vi "measure_max_power_stabilisation_keithley-2400.vi"(0 "User Name":string, 1 "Cell details cluster":T2={"Cell Position"=16, "Cell Label"="", "Pixel to measure"=0, "Area (cm^2)"=0.126, "Variable"="", "Variable value"="", "Scan settings in queue"=0, "Light or dark"="", "Measurement Type"=""} {"Pixel to measure" items=["All", "1", "2", "3", "4", "5", "6", "7", "8"]}, 3 "Date array":string[](array[string]), 5 "Experiment Title":string, 9 "File path of JV log":path, 11 "Intensity (no. of suns)":string, 12 "Scan settings":T1={"J-V scan"=TRUE, "Start voltage (V)"=0.0, "End voltage (V)"=0.0, "Step voltage (V)"=1.4, "Scan both directions"=TRUE, "Inverted device structure"=FALSE, "Settling delay (ms)"=10.0, "Measurement speed"=0, "Scan rate (V/s)"=0.0, "Stabilisation time (s)"=0.0, "Stabilisation mode"=0, "Stabilisation value (V or A) "=1.0, "Illumination"=0, "Stabilisation in the dark?"=FALSE, "Repeat light scans"=FALSE, "No. of repeat scans"=0.0, "Only repeat for best pixel"=1, "J-t scan"=FALSE, "J-t best pixel only"=7, "J-t start voltage (V)"=0.0, "J-t end voltage (V)"=1.4, "J-t step voltage (V)"=0.01, "Step time (s)"=0.7, "J-t scan both directions"=TRUE, "J-t inverted device structure"=FALSE, "J-t settling delay (ms)"=0.0, "J-t measurement speed"=0, "J-t illumination"=2, "Max. power stabilisation"=FALSE, "Max power best pixel only"=1, "Max. power point tracker"=FALSE, "Vmp from J-V scan"=FALSE, "Max P stab. Specific voltage"=FALSE, "Vmp (V)"=1.0, "Stabilisation time step (s)"=1.0, "Total stabilisation time (s)"=100.0} {"J-t settling delay (ms)" min=10.0; "J-t illumination" items=["Light only", "Dark only", "Light then dark", "Dark then light"]; "Measurement speed" items=["Fast", "Normal", "High accuracy"]; "Illumination" items=["Light only", "Dark only", "Light then dark", "Dark then light"]; "Only repeat for best pixel" items=["only for best pixel", "for best 2 pixels", "for best 3 pixels", "for best 4 pixels", "for best 5 pixels", "for best 6 pixels", "for best 7 pixels", "for all pixels"]; "No. of repeat scans" min=1.0 step=1.0; "Max power best pixel only" items=["only the best pixel", "the best 2 pixels", "the best 3 pixels", "the best 4 pixels", "the best 5 pixels", "the best 6 pixels", "the best 7 pixels", "all pixels"]; "J-t best pixel only" items=["only the best pixel", "the best 2 pixels", "the best 3 pixels", "the best 4 pixels", "the best 5 pixels", "the best 6 pixels", "the best 7 pixels", "all pixels"]; "J-t measurement speed" items=["Fast", "Normal", "High Accuracy"]; "Stabilisation mode" items=["V", "I"]; "Settling delay (ms)" min=10.0}, 13 "VISA resource name":refnum<visa-resource-name>="GPIB1::24::INSTR", 14 "Skip pixel?":bool) -> (4 "Jt Curve":cluster{"Y":dbl[], "Y":dbl[]}[](graph) caption="JV Curve")   [LabVIEW 2016]
uses:
  TypeDefs/scan_settings.ctl
  <vilib>/Utility/file.llb/Read Delimited Spreadsheet (DBL).vi
  <instrlib>/Keithley 24XX/Keithley 24XX.lvlib
panel:
  out "File path for Jt image":path
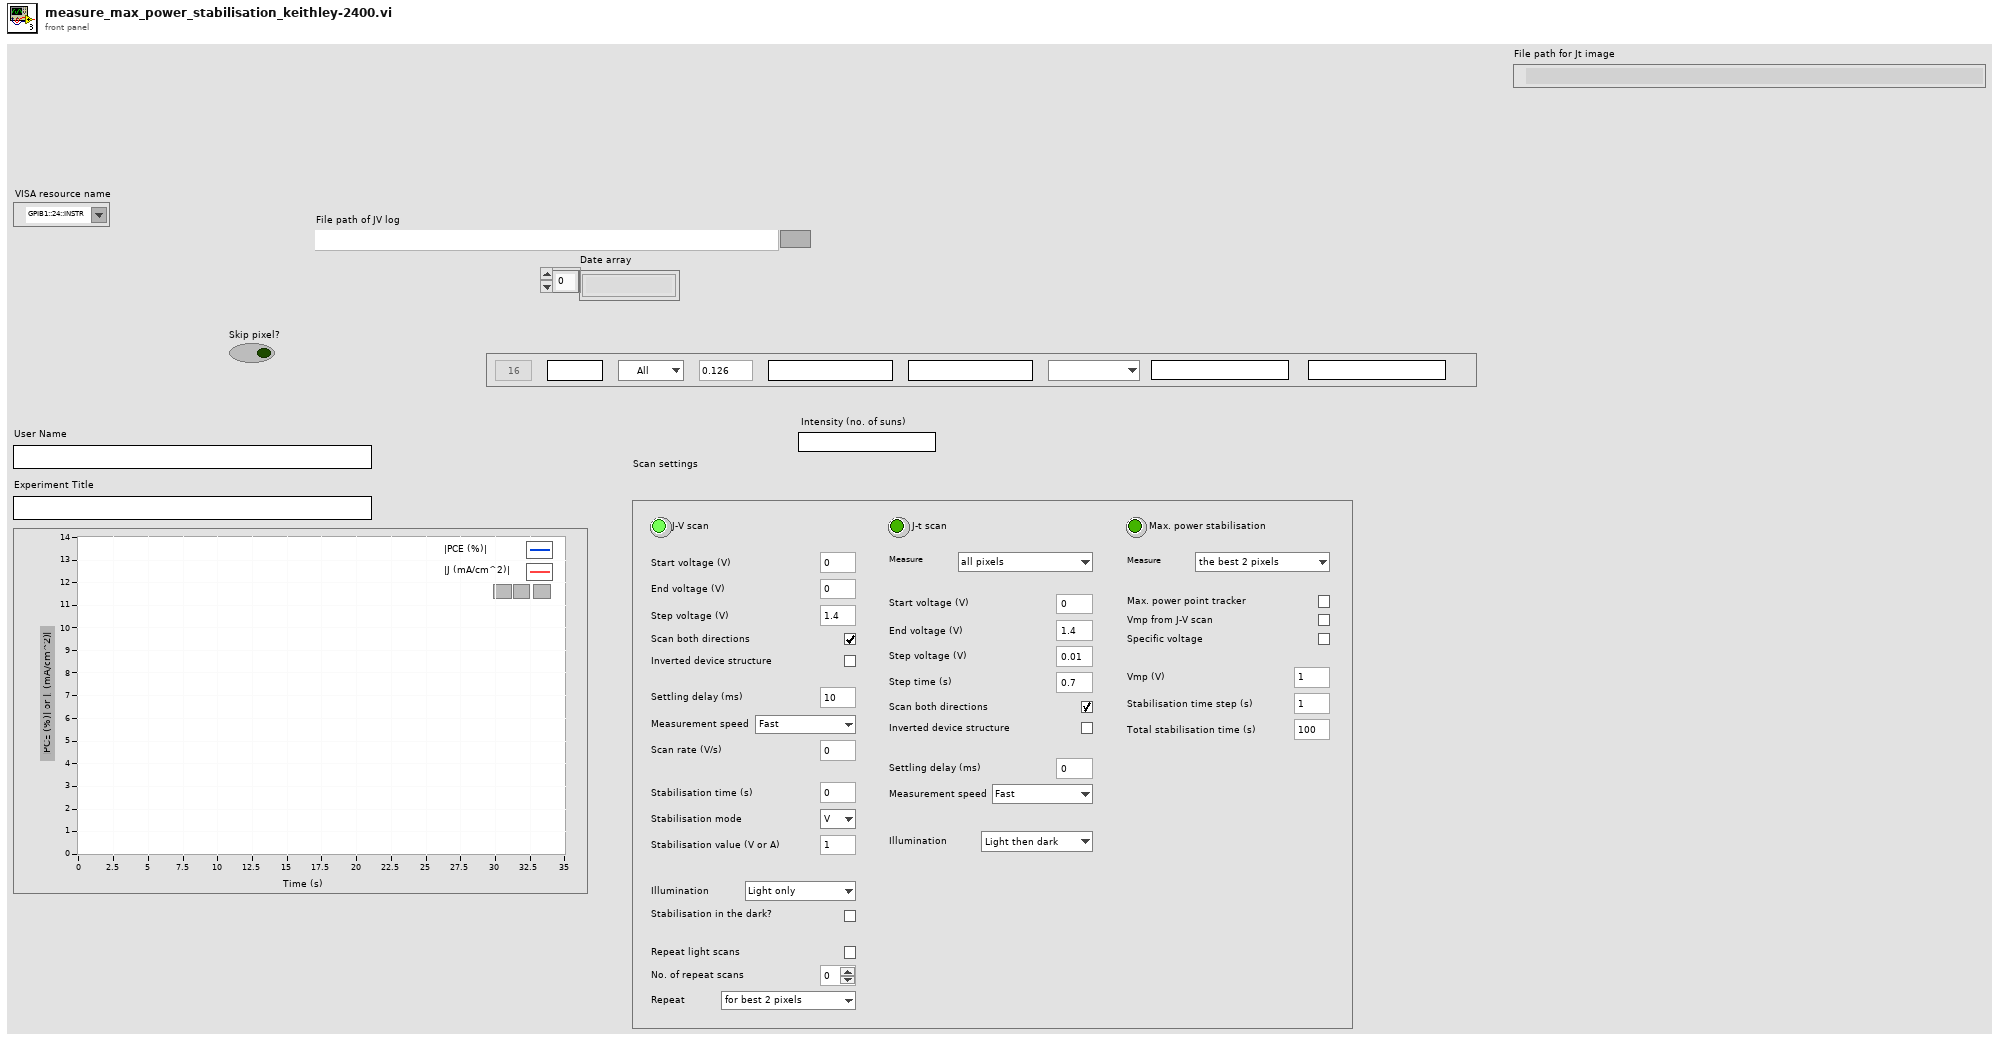
[diagram p1: front panel]
types:
  T1 = typedef "scan_settings.ctl" = cluster{"J-V scan":bool, "Start voltage (V)":dbl, "End voltage (V)":dbl, "Step voltage (V)":dbl, "Scan both directions":bool, "Inverted device structure":bool, "Settling delay (ms)":dbl, "Measurement speed":u8, "Scan rate (V/s)":dbl, "Stabilisation time (s)":dbl, "Stabilisation mode":u16, "Stabilisation value (V or A) ":dbl, "Illumination":u16, "Stabilisation in the dark?":bool, "Repeat light scans":bool, "No. of repeat scans":dbl, "Only repeat for best pixel":u16, "J-t scan":bool, "J-t best pixel only":u16, "J-t start voltage (V)":dbl, "J-t end voltage (V)":dbl, "J-t step voltage (V)":dbl, "Step time (s)":dbl, "J-t scan both directions":bool, "J-t inverted device structure":bool, "J-t settling delay (ms)":dbl, "J-t measurement speed":u16, "J-t illumination":u16, "Max. power stabilisation":bool, "Max power best pixel only":u16, "Max. power point tracker":bool, "Vmp from J-V scan":bool, "Max P stab. Specific voltage":bool, "Vmp (V)":dbl, "Stabilisation time step (s)":dbl, "Total stabilisation time (s)":dbl}
  T2 = cluster{"Cell Position":i32, "Cell Label":string, "Pixel to measure":u16, "Area (cm^2)":dbl, "Variable":string, "Variable value":string, "Scan settings in queue":u16, "Light or dark":string, "Measurement Type":string}
  T3 = typedef "imagedata.ctl" = cluster{"image type":i32, "image depth":i32, "image":u8[], "mask":u8[], "colors":u32[], "Rectangle":cluster{"left":i16, "top":i16, "right":i16, "bottom":i16}}
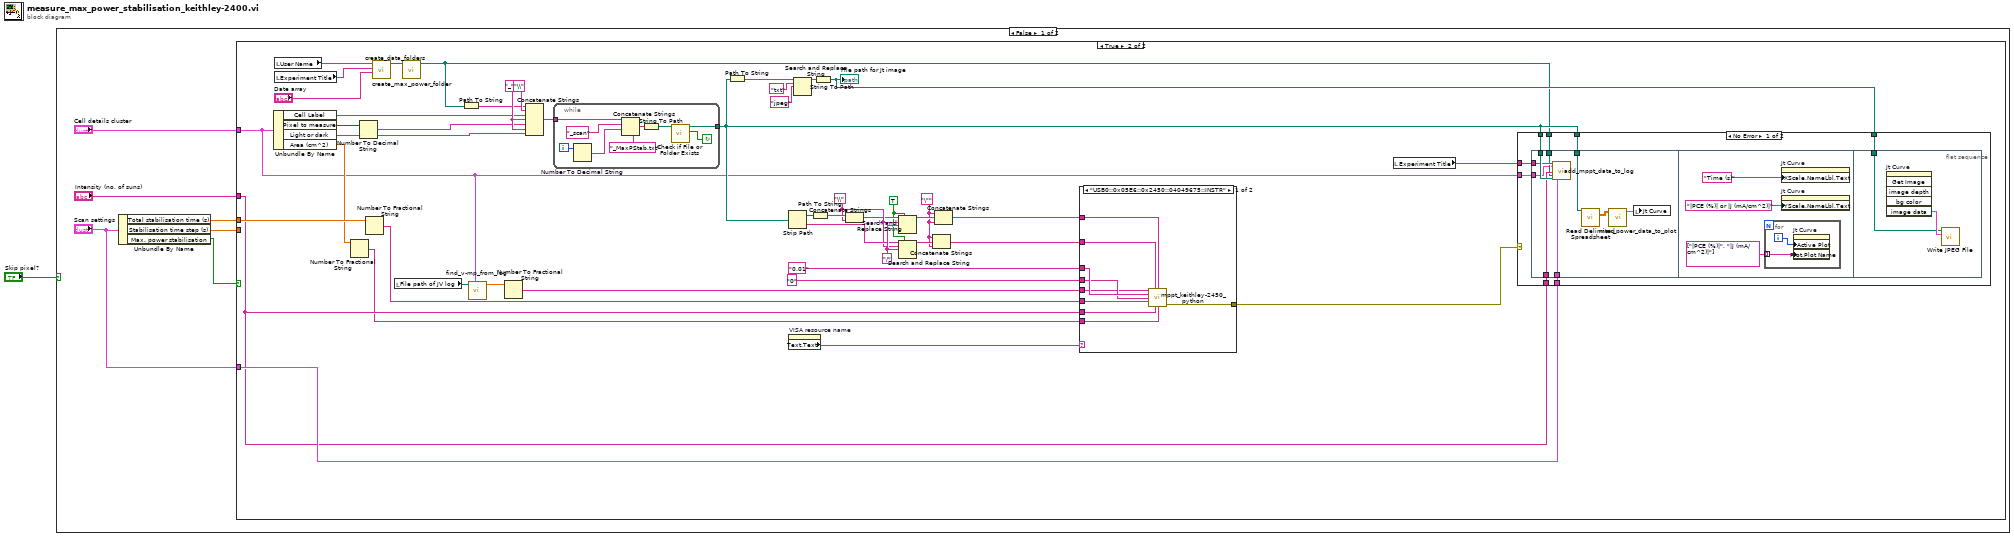
[diagram p0: block diagram]
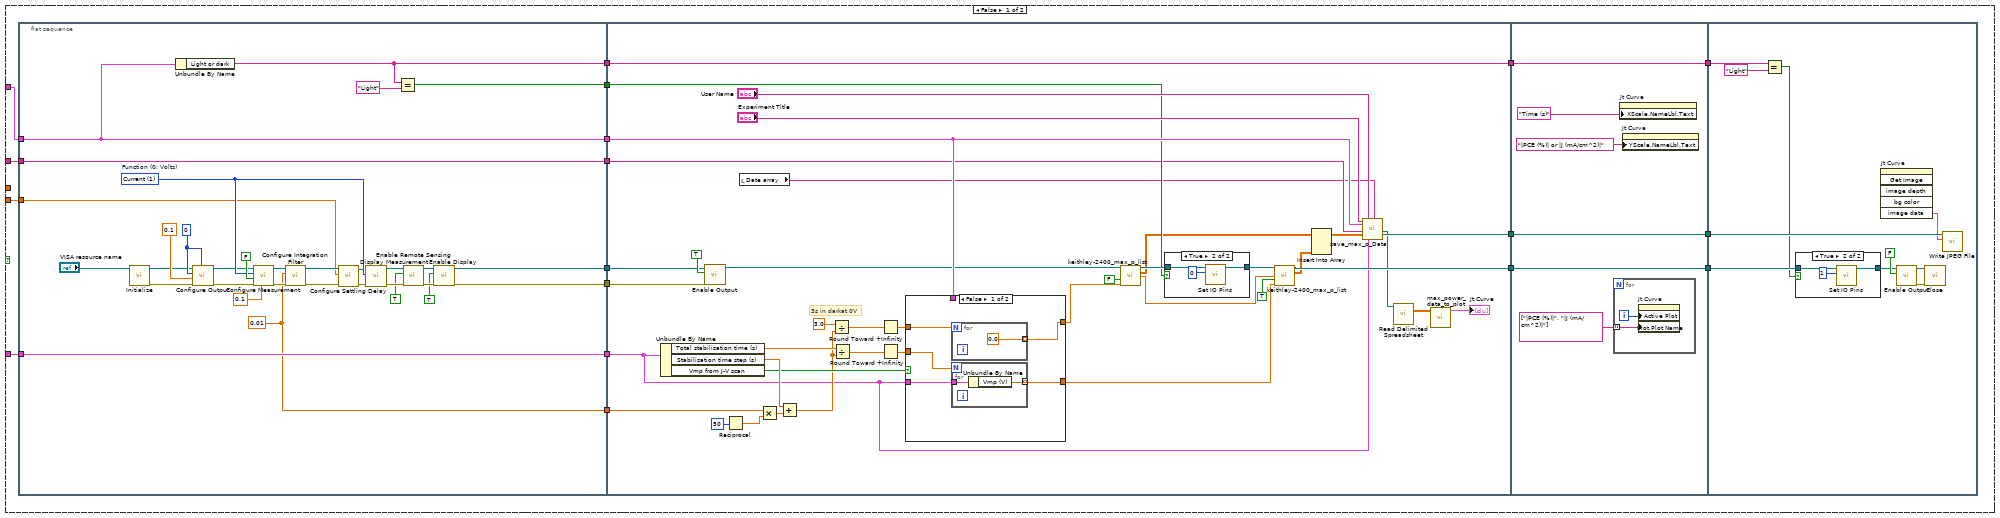
[diagram p2: hidden frame]
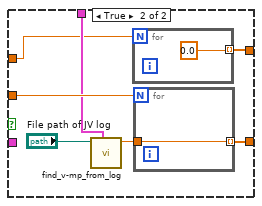
[diagram p4: hidden frame]
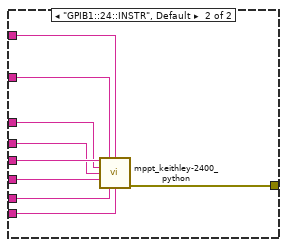
[diagram p6: hidden frame]
diagram:
  n1 = case shown="False" "Skip pixel?" {
    frame False {
      n2 = Unbundle By Name("Scan settings") -> ("Total stabilisation time (s)"=w3:dbl, "Stabilisation time step (s)"=w7:dbl, "Max. power stabilisation"=w4:bool)
      n3 = case shown="True" w4 {
        tunnel: w7 -> [w18 _]
        tunnel: "Cell details cluster" -> [w17 w155]
        tunnel: "Scan settings" -> [w16 w159]
        tunnel: w3 -> [_ w167]
        tunnel: "Intensity (no. of suns)" -> [w14 w151]
        frame False {
          n4 = flat-sequence {
            tunnel: [w35] -> w24
            tunnel: [w36] -> w25
            tunnel: [w37] -> w23
            tunnel: w18 -> [w38]
            tunnel: [w40] -> w22
            tunnel: w17 -> [w40]
            tunnel: [w42] -> w21
            tunnel: w16 -> [w42]
            tunnel: [w39] -> w20
            tunnel: [w34] -> w19
            tunnel: [w26] -> w15
            tunnel: w14 -> [w26]
            tunnel: [w95] -> w13
            tunnel: [w97] -> w11
            tunnel: w25 -> [w64]
            tunnel: w24 -> [w63]
            tunnel: w23 -> [w88]
            tunnel: w22 -> [w81]
            tunnel: w21 -> [w58]
            tunnel: [w91] -> w9
            tunnel: w20 -> [w91]
            tunnel: w19 -> [w68]
            tunnel: w15 -> [w62]
            tunnel: w13 -> [w124]
            tunnel: [w124] -> w12
            tunnel: w11 -> [w123]
            tunnel: [w123] -> w10
            tunnel: w9 -> [w122]
            tunnel: [w122] -> w8
            tunnel: w12 -> [w130]
            tunnel: w10 -> [w133]
            tunnel: w8 -> [w127]
            frame #0 {
              w32 = 0
              w37 = 0.01
              w48 = u16 1 items=["Volts", "Current", "Resistance"]  # Function (0: Volts)
              n5 = call <instrlib>:"Initialize.vi"("VISA resource name"="VISA resource name") -> ("error out"=w27:errorcluster, "VISA resource name out"=w30:refnum<visa-resource-name>)  [unwired: 4 in, 5 out]
              n6 = Unbundle By Name(w40) -> ("Light or dark"=w39:string)
              n7 = call <instrlib>:"Configure Output.vi"("Source Mode  (0: Voltage)"=w32, "error in (no error)"=w27, "Compliance  Level (0.1)"=0.1, "Output Level (0)"=w32, "VISA resource name"=w30) -> ("error out"=w28:errorcluster, "VISA resource name out"=w29:refnum<visa-resource-name>)  [unwired: 5 in]
              n8 = call <instrlib>:"Configure Measurement.vi"("Manual Range (1.0)"=0.1, "error in (no error)"=w28, "Enable Auto Range (T:Enable)"=FALSE, "Function (0: Volts)"=w48, "VISA resource name"=w29) -> ("error out"=w53:errorcluster, "VISA resource name out"=w52:refnum<visa-resource-name>)  [unwired: 5 in]
              n9 = call <instrlib>:"Configure Integration Filter.vi"("error in (no error)"=w53, "Measurement Speed (1 PLC)"=w37, "VISA resource name"=w52) -> ("error out"=w43:errorcluster, "VISA resource name out"=w46:refnum<visa-resource-name>)  [unwired: 7 in]
              n10 = call <instrlib>:"Configure Settling Delay.vi"("error in (no error)"=w43, "Manual Settling Delay (0 sec)"=w38, "VISA resource name"=w46) -> ("error out"=w44:errorcluster, "VISA resource name out"=w45:refnum<visa-resource-name>)  [unwired: 7 in]
              n11 = call <instrlib>:"Display Measurement.vi"("error in (no error)"=w44, "Displayed Measurement (0: Voltage)"=w48, "VISA resource name"=w45) -> ("error out"=w55:errorcluster, "VISA resource name out"=w54:refnum<visa-resource-name>)  [unwired: 7 in]
              n12 = Equal?(x=w39, y="Light") -> (x = y?=w34:bool)
              n13 = call <instrlib>:"Enable Remote Sensing.vi"("error in (no error)"=w55, "Enable Remote Sensing (T: Enable)"=TRUE ("Enable Output (T: Enable)"), "VISA resource name"=w54) -> ("error out"=w50:errorcluster, "VISA resource name out"=w51:refnum<visa-resource-name>)  [unwired: 7 in]
              n14 = call <instrlib>:"Enable Display.vi"("error in (no error)"=w50, "Enable Display (T: Enable)"=TRUE ("Enable Output (T: Enable)"), "VISA resource name"=w51) -> ("error out"=w35:errorcluster, "VISA resource name out"=w36:refnum<visa-resource-name>)  [unwired: 7 in]
            }
            frame #1 {
              # "3s in darkat 0V"
              n15 = Unbundle By Name(w58) -> ("Total stabilisation time (s)"=w85:dbl, "Stabilisation time step (s)"=w86:dbl, "Vmp from J-V scan"=w82:bool)
              n16 = call <instrlib>:"Enable Output.vi"("error in (no error)"=w63, "Enable Output (T: Enable)"=TRUE ("Output (Off)"), "VISA resource name"=w64) -> ("VISA resource name out"=w73:refnum<visa-resource-name>)  [unwired: 7 in, 1 out]
              n17 = Reciprocal(x=50) -> (1/x=w90:dbl)
              n18 = local read "Date array"() -> (w59:string[])
              n19 = Multiply(x=w88, y=w90) -> (x*y=w87:dbl)
              n20 = Add(x=w86, y=w87) -> (x+y=w80:dbl)
              n21 = Divide(x=3.0, y=w80) -> (x/y=w77:dbl)
              n22 = Divide(x=w85, y=w80) -> (x/y=w78:dbl)
              n23 = Round Toward +Infinity(x=w77) -> (ceil(x): smallest int >= x=w76:dbl)
              n24 = Round Toward +Infinity(x=w78) -> (ceil(x): smallest int >= x=w84:dbl)
              n25 = case shown="False" w82 {
                tunnel: w84 -> [w106 w115]
                tunnel: w58 -> [w104 _]
                tunnel: [w105 w114] -> w83
                tunnel: w81 -> [_ w113]
                tunnel: w76 -> [w103 w112]
                tunnel: [w102 w111] -> w74
                frame False {
                  n26 = for {
                    N: w103 -> [_]
                    tunnel: [0.0 ("Vmp")] -> w102 mode=indexing
                  }
                  n27 = for {
                    N: w106 -> [_]
                    tunnel: w104 -> [w109]
                    tunnel: [w108] -> w105 mode=indexing
                    n28 = Unbundle By Name(w109) -> ("Vmp (V)"=w108:dbl)
                  }
                }
                frame True {
                  n29 = call "find_v-mp_from_log.vi"("Cell details cluster in"=w113, "File path of JV log"="File path of JV log") -> ("Vmp"=w110:dbl)  [unwired: 9 in]
                  n30 = for {
                    N: w112 -> [_]
                    tunnel: [0.0 ("Vmp")] -> w111 mode=indexing
                  }
                  n31 = for {
                    N: w115 -> [_]
                    tunnel: [w118] -> w114 mode=indexing
                    tunnel: w110 -> [w118]
                  }
                }
              }
              n32 = call "keithley-2400_max_p_list.vi"("VISA resource name in"=w73, "Light?"=FALSE, "Voltage List"=w74) -> ("VISA resource name out"=w70:refnum<visa-resource-name>, "Data Array"=w67:dbl[][], "timestamp"=w69:sgl)  [unwired: 9 in, 1 out]
              n33 = case shown="True" w68 {
                tunnel: w70 -> [w98 w100]
                tunnel: [w98 w99] -> w75
                frame False {
                }
                frame True {
                  n34 = call <instrlib>:"Set IO Pins.vi"("Output Pattern (0)"=0, "VISA resource name"=w100) -> ("VISA resource name out"=w99:refnum<visa-resource-name>)  [unwired: 8 in, 1 out]
                }
              }
              n35 = call "keithley-2400_max_p_list.vi"("VISA resource name in"=w75, "t=0 timestamp"=w69, "Light?"=TRUE, "Voltage List"=w83) -> ("VISA resource name out"=w95:refnum<visa-resource-name>, "Data Array"=w66:dbl[][])  [unwired: 8 in, 2 out]
              n36 = Insert Into Array(array=w67, new element=w66) -> (w65:dbl[][])  [unwired: 2 in]
              n37 = call "save_max_p_Data.vi"("Experiment Indicator"="Experiment Title", "Cell details cluster"=w81, "Intensity (no. of suns)"=w62, "Data Array"=w65, "Username"="User Name", "Scan settings"=w58, "Date array"=w59) -> ("File path for Jt data"=w61:path, "File path for Jt image"=w97:path)  [unwired: 9 in, 2 out]
              n38 = call-poly <vilib>:"Read Delimited Spreadsheet.vi"("file path (dialog if empty)"=w61) -> ("all rows"=w60:dbl[][])  [unwired: 9 in, 5 out]
              n39 = call "max_power_data_to_plot.vi"("Data Array"=w60) -> ("JV Curve"=→"Jt Curve":cluster{"Y":dbl[], "Y":dbl[]}[])  [unwired: 10 in]
            }
            frame #2 {
              n40 = for {
                tunnel: string[] ["|PCE (%)|", "|J (mA/cm^2)|"] ("Measurement queue") -> [w125] mode=indexing
                i -> [w126]
                n41 = property on="Jt Curve" class="XYGraph (strict)"("Active Plot"=w126, "Plot.Plot Name"=w125) -> ()  [unwired: 2 in, 2 out]
              }
              n42 = property on="Jt Curve" class="XYGraph (strict)"("XScale.NameLbl.Text"="Time (s)" ("Y Scale.Name Label.Text")) -> ()  [unwired: 2 in, 2 out]
              n43 = property on="Jt Curve" class="XYGraph (strict)"("YScale.NameLbl.Text"="|PCE (%)| or |J (mA/cm^2)|" ("Y Scale.Name Label.Text")) -> ()  [unwired: 2 in, 2 out]
            }
            frame #3 {
              n44 = Equal?(x=w127, y="Light") -> (x = y?=w128:bool)
              n45 = case shown="True" w128 {
                tunnel: w130 -> [w137 w139]
                tunnel: [w137 w138] -> w129
                frame False {
                }
                frame True {
                  n46 = call <instrlib>:"Set IO Pins.vi"("Output Pattern (0)"=1, "VISA resource name"=w139) -> ("VISA resource name out"=w138:refnum<visa-resource-name>)  [unwired: 8 in, 1 out]
                }
              }
              n47 = invoke on="Jt Curve" class="XYGraph (strict)" method="Get Image"() -> ("image data"=w132:T3)  [unwired: 6 in, 5 out]
              n48 = call <instrlib>:"Enable Output.vi"("Enable Output (T: Enable)"=FALSE ("Output (Off)"), "VISA resource name"=w129) -> ("error out"=w135:errorcluster, "VISA resource name out"=w136:refnum<visa-resource-name>)  [unwired: 8 in]
              n49 = call <instrlib>:"Close.vi"("error in (no error)"=w135, "VISA resource name"=w136) -> ()  [unwired: 9 in, 1 out]
              n50 = call <vilib>:"Write JPEG File.vi"("image data"=w132, "path to JPEG file"=w133) -> ()  [unwired: 8 in, 2 out]
            }
          }
        }
        frame True {
          w154 = "\"" ("string")
          w142 = TRUE ("replace all? (F)")
          w170 = "/" ("search string")
          w153 = "\\" ("search string")
          w179 = "_"
          n51 = Unbundle By Name(w155) -> ("Cell Label"=w175:string, "Pixel to measure"=w176:u16, "Light or dark"=w173:string, "Area (cm^2)"=w164:dbl)
          n52 = local read "User Name"() -> (w181:string)
          n53 = local read "Experiment Title"() -> (w182:string)
          n54 = Number To Fractional String(number=w164) -> (F-format string=w150:string)  [unwired: 3 in]
          n55 = Number To Decimal String(number=w176) -> (decimal integer string=w174:string)  [unwired: 1 in]
          n56 = Number To Fractional String(number=w167) -> (F-format string=w149:string)  [unwired: 3 in]
          n57 = call "create_data_folders.vi"("Date array"="Date array", "Experiment Indicator"=w182, "username"=w181) -> ("Data Output Folder"=w180:path)  [unwired: 8 in]
          n58 = local read "File path of JV log"() -> (w166:path)
          n59 = call "create_max_power_folder.vi"("Data Folder In"=w180) -> ("Data Output Folder"=w156:path)  [unwired: 10 in]
          n60 = Path To String(path=w156) -> (string=w171:string)
          n61 = call "find_v-mp_from_log.vi"("Cell details cluster in"=w155, "File path of JV log"=w166) -> ("Vmp"=w165:dbl)  [unwired: 9 in]
          n62 = Number To Fractional String(number=w165) -> (F-format string=w148:string)  [unwired: 3 in]
          n63 = Concatenate Strings(w171, "\\", w175, w179, w174, w179, w173) -> (w178:string)
          n64 = while {
            tunnel: w178 -> [w237]
            tunnel: [w229] -> w158
            i -> [w235]
            stop <- w230 continue-if-true
            n65 = Number To Decimal String(number=w235) -> (decimal integer string=w234:string)  [unwired: 1 in]
            n66 = Concatenate Strings(w237, "_scan", w234, "_MaxPStab.txt") -> (w231:string)
            n67 = String To Path(string=w231) -> (path=w232:path)
            n68 = call <vilib>:"Check if File or Folder Exists.vi"("path"=w232) -> ("file or folder exists?"=w230:bool, "dup path"=w229:path)  [unwired: 8 in, 1 out]
          }
          n69 = Path To String(path=w158) -> (string=w186:string)
          n70 = Strip Path(path=w158) -> (stripped path=w162:path, name=w163:string)
          n71 = property on="VISA resource name" class="VISAName"() -> ("Text.Text"=w141:string)  [unwired: 2 in, 2 out]
          n72 = Search and Replace String(input string=w186, search string="txt", replace string="jpeg") -> (result string=w183:string)  [unwired: 5 in, 3 out]
          n73 = Path To String(path=w162) -> (string=w161:string)
          n74 = String To Path(string=w183) -> (path=w168:path)
          "File path for Jt image" <- w168
          n75 = Concatenate Strings(w161, w153) -> (w143:string)
          n76 = Search and Replace String(replace all?=w142, input string=w163, search string=w153, replace string=w170) -> (result string=w169:string)  [unwired: 4 in, 3 out]
          n77 = Search and Replace String(replace all?=w142, input string=w143, search string=w153, replace string=w170) -> (result string=w172:string)  [unwired: 4 in, 3 out]
          n78 = Concatenate Strings(w154, w169, w154) -> (w146:string)
          n79 = Concatenate Strings(w154, w172, w154) -> (w147:string)
          n80 = case shown="\"USB0::0x05E6::0x2450::04049675::INSTR\"" w141 {
            tunnel: [w195 w204] -> w152
            tunnel: w151 -> [w188 w203]
            tunnel: w150 -> [w187 w202]
            tunnel: w149 -> [w189 w201]
            tunnel: w148 -> [w190 w200]
            tunnel: w147 -> [w194 w199]
            tunnel: w146 -> [w193 w198]
            tunnel: "0.01" ("search string") -> [w192 w197]
            tunnel: "0" ("search string") -> [w191 w196]
            frame "USB0::0x05E6::0x2450::04049675::INSTR" {
              n81 = call "mppt_keithley-2450_python.vi"("start voltage (V)"=w190, "file name"=w193, "folder path"=w194, "nplc"=w192, "settling delay (s)"=w191, "total tracking time (s)"=w189, "illumination intensity (suns equiv.)"=w188, "area (cm^2)"=w187) -> ("error out"=w195:errorcluster)  [unwired: 7 in]
            }
            frame "GPIB1::24::INSTR", Default {
              n82 = call "mppt_keithley-2400_python.vi"("start voltage (V)"=w200, "file name"=w198, "folder path"=w199, "nplc"=w197, "settling delay (s)"=w196, "total tracking time (s)"=w201, "illumination intensity (suns equiv.)"=w203, "area (cm^2)"=w202) -> ("error out"=w204:errorcluster)  [unwired: 7 in]
            }
          }
          n83 = local read "Experiment Title"() -> (w157:string)
          n84 = case shown="No Error" w152 {
            tunnel: w158 -> [w212 _]
            tunnel: w168 -> [w211 _]
            tunnel: w159 -> [w210 _]
            tunnel: w158 -> [w209 _]
            tunnel: w151 -> [w208 _]
            tunnel: w157 -> [w207 _]
            tunnel: w156 -> [w206 _]
            tunnel: w155 -> [w205 _]
            frame No Error {
              n85 = flat-sequence {
                tunnel: w212 -> [w221]
                tunnel: w210 -> [w218]
                tunnel: w209 -> [w217]
                tunnel: w208 -> [w216]
                tunnel: w207 -> [w215]
                tunnel: w206 -> [w214]
                tunnel: w205 -> [w213]
                tunnel: w211 -> [w227]
                frame #0 {
                  n86 = call "add_mppt_data_to_log.vi"("Experiment Indicator"=w215, "Cell details cluster"=w213, "Intensity (no. of suns)"=w216, "mppt folder path"=w214, "mppt file path"=w217, "Scan settings"=w218) -> ()  [unwired: 12 in, 2 out]
                  n87 = call-poly <vilib>:"Read Delimited Spreadsheet.vi"("file path (dialog if empty)"=w221) -> ("all rows"=w220:dbl[][])  [unwired: 9 in, 5 out]
                  n88 = call "max_power_data_to_plot.vi"("Data Array"=w220) -> ("JV Curve"=w219:cluster{"Y":dbl[], "Y":dbl[]}[])  [unwired: 10 in]
                  n89 = local write "Jt Curve"(w219) -> ()
                }
                frame #1 {
                  n90 = for {
                    tunnel: string[] ["|PCE (%)|", "|J (mA/cm^2)|"] ("Measurement queue") -> [w225] mode=indexing
                    i -> [w226]
                    n91 = property on="Jt Curve" class="XYGraph (strict)"("Active Plot"=w226, "Plot.Plot Name"=w225) -> ()  [unwired: 2 in, 2 out]
                  }
                  n92 = property on="Jt Curve" class="XYGraph (strict)"("XScale.NameLbl.Text"="Time (s)" ("Y Scale.Name Label.Text")) -> ()  [unwired: 2 in, 2 out]
                  n93 = property on="Jt Curve" class="XYGraph (strict)"("YScale.NameLbl.Text"="|PCE (%)| or |J (mA/cm^2)|" ("Y Scale.Name Label.Text")) -> ()  [unwired: 2 in, 2 out]
                }
                frame #2 {
                  n94 = invoke on="Jt Curve" class="XYGraph (strict)" method="Get Image"() -> ("image data"=w228:T3)  [unwired: 6 in, 5 out]
                  n95 = call <vilib>:"Write JPEG File.vi"("image data"=w228, "path to JPEG file"=w227) -> ()  [unwired: 8 in, 2 out]
                }
              }
            }
            frame Error {
            }
          }
        }
      }
    }
    frame True {
    }
  }
